vi "AccelePID.vi"(4 "Top Speed":dbl, 5 "Acceleration Rate":dbl, 6 "reinitialize? (F)":bool, 7 "output range":cluster{"output high":dbl, "output low":dbl}={"output high"=100.0, "output low"=-100.0} {"output low" format="%.2f"; "output high" format="%.2f"}, 8 "dt (s)":dbl=-1.0 format="%.3f", 9 "PID gains":T1={"proportional gain (Kc)"=1.0, "integral time (Ti, min)"=0.01, "derivative time (Td, min)"=0.0} {"derivative time (Td, min)" format="%.3f"; "integral time (Ti, min)" format="%.3f"; "proportional gain (Kc)" format="%.3f"}, 10 "process variable":dbl format="%.2f", 11 "setpoint":dbl format="%.2f") -> (0 "dt out (s)":dbl format="%.3f", 2 "output":dbl format="%.2f")   [LabVIEW 2013]
uses:
  <vilib>/addons/control/pid/pid.llb/PID (DBL).vi
  <vilib>/addons/control/pid/NI_PID_pid.lvlib
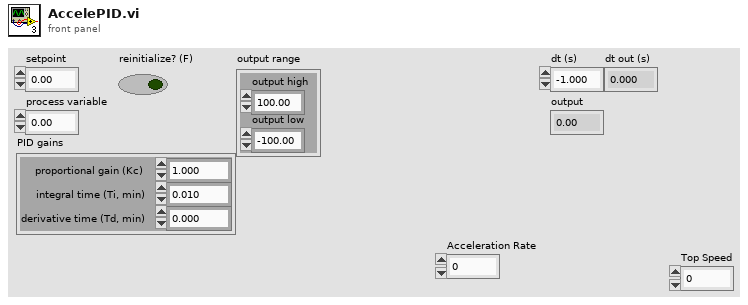
[diagram p1: front panel]
types:
  T1 = cluster{"proportional gain (Kc)":dbl, "integral time (Ti, min)":dbl, "derivative time (Td, min)":dbl}
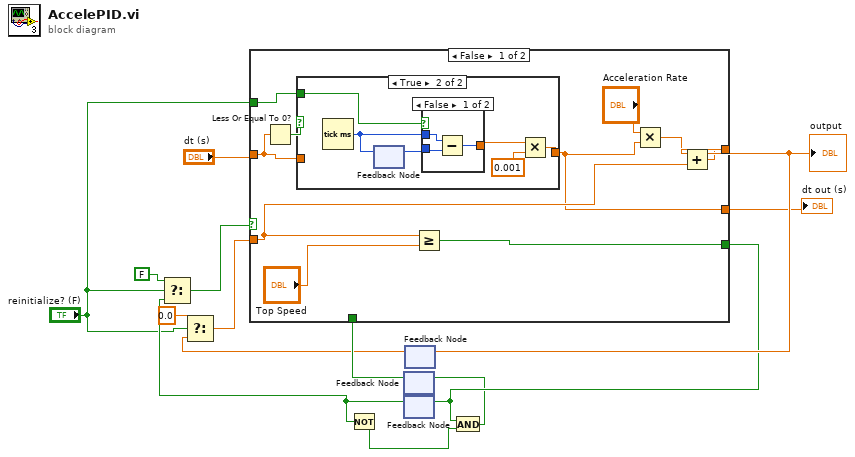
[diagram p0: block diagram]
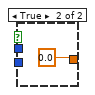
[diagram p3: hidden frame]
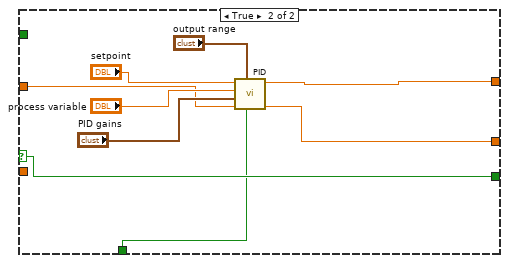
[diagram p4: hidden frame]
diagram:
  n1 = feedback #1() -> (w8:bool)  [unwired: 1 in]
  n2 = feedback #2() -> (w5:bool)  [unwired: 1 in]
  n3 = Select(t=FALSE, s="reinitialize? (F)", f=w5) -> (s? t:f=w4:bool)
  n4 = Not(x=w5) -> (.not. x?=w10:bool)
  n5 = feedback #3() -> (w7:dbl)  [unwired: 1 in]
  n6 = Select(t=0.0, s="reinitialize? (F)", f=w7) -> (s? t:f=w6:dbl)
  n7 = case shown="False" w4 {
    selector: w4 -> [_ w37]
    tunnel: [w19 w41] -> w14
    tunnel: "dt (s)" -> [w17 w39]
    tunnel: [w15 w38] -> w12
    tunnel: w6 -> [w20 _]
    tunnel: [w23 w37] -> w11
    tunnel: w8 -> [_ w36]
    tunnel: "reinitialize? (F)" -> [w16 _]
    frame False {
      n8 = Less Or Equal To 0?(x=w17) -> (x <= 0?=w18:bool)
      n9 = case shown="True" w18 {
        tunnel: w17 -> [w25 _]
        tunnel: [w25 w27] -> w15
        tunnel: w16 -> [_ w26]
        frame False {
        }
        frame True {
          n10 = Tick Count (ms)() -> (millisecond timer value=w31:u32)
          n11 = feedback #4() -> (w30:u32)  [unwired: 1 in]
          n12 = feedback-in #4(w31) -> ()
          n13 = case shown="False" w26 {
            tunnel: w30 -> [w32 _]
            tunnel: w31 -> [w33 _]
            tunnel: [w34 0.0] -> w28
            frame False {
              n14 = Subtract(x=w33, y=w32) -> (x-y=w34:u32)
            }
            frame True {
            }
          }
          n15 = Multiply(x=w28, y=0.001) -> (x*y=w27:dbl)
        }
      }
      n16 = Greater Or Equal?(x=w20, y="Top Speed") -> (x >= y?=w23:bool)
      n17 = Multiply(x="Acceleration Rate", y=w15) -> (x*y=w21:dbl)
      n18 = Add(x=w21, y=w20) -> (x+y=w19:dbl)
    }
    frame True {
      n19 = call-poly <vilib>:"PID.vi"("reinitialize? (F)"=w36, "output range"="output range", "dt (s)"=w39, "PID gains"="PID gains", "process variable"="process variable", "setpoint"="setpoint") -> ("dt out (s)"=w38:dbl, "output"=w41:dbl)  [unwired: 4 in]
    }
  }
  "output" <- w14
  "dt out (s)" <- w12
  n20 = feedback-in #2(w11) -> ()
  n21 = feedback-in #3(w14) -> ()
  n22 = And(x=w11, y=w10) -> (x .and. y?=w9:bool)
  n23 = feedback-in #1(w9) -> ()
